vi "Do.vi"(8 "error in":errorcluster, 10 "Actor in":refnum<class "Actor.lvclass">, 11 "Enable Laser Channel 0":refnum<class "Update PAS Laser 0 Enable State MSG.lvclass">) -> (0 "error out":errorcluster, 2 "Actor out":refnum<class "Actor.lvclass">)   [LabVIEW 2016, in "Controller.lvlib" / "Update PAS Laser 0 Enable State MSG.lvclass"]
doc: "(<B>Filename</B>: Actor Framework.lvlib:Message.lvclass:Do.vi)\n\nDefines what a message does when it is received by an actor. Generally, a message instructs an actor to invoke one of its methods. By default, this method does nothing. A child class must override it to define behavior. Create a child class by using the Actor Framework Message Maker dialog box."
uses:
  Update PAS Laser 0 Enable State MSG.lvclass
  G:/sw_repo/For Builds/Nicholas/Controller/Messages/Generic Boolean MSG/Generic Boolean Message.lvclass
  <vilib>/ActorFramework/Actor/Actor.lvclass
  Generic Boolean MSG/Generic Boolean Message.lvclass/Generic Boolean Message.ctl
  Generic Boolean MSG/Read Bool.vi
  <vilib>/rvi/errors/niLvFpgaAdjustHostInterfaceError.vi
  <vilib>/Utility/error.llb/Error Cluster From Error Code.vi
  FPGA Ref.ctl
  <vilib>/rvi/interface/nirviReadWriteControl/nirviReadWriteControl.xnode
  FPGA Bitfiles/serverv4.lvbitx
  gController.lvclass
  NiFpgaLv.dll
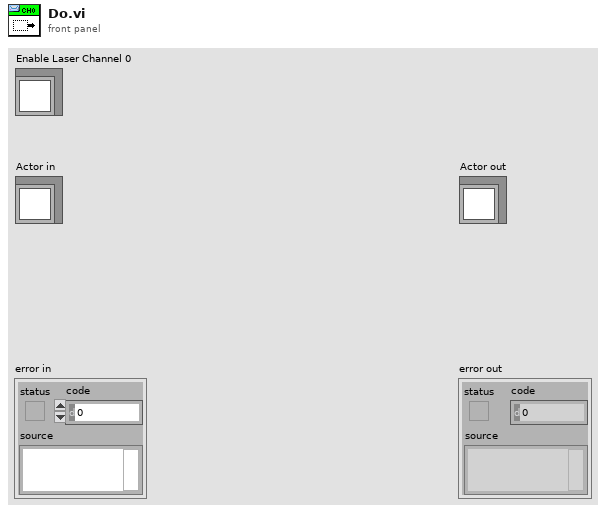
[diagram p1: front panel]
types:
  T1 = typedef "FPGA Ref.ctl" = refnum<k20>
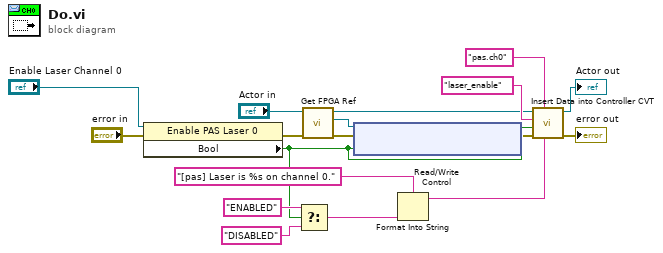
[diagram p0: block diagram]
diagram:
  n1 = property class="Enable PAS Laser 0"(reference="Enable Laser Channel 0", error in="error in") -> (error out=w4:errorcluster, "Bool"=w5:bool)  [unwired: 1 out]
  n2 = Select(t="ENABLED", s=w5, f="DISABLED") -> (s? t:f=w11:string)
  n3 = call "Get FPGA Ref.vi"("error in (no error)"=w4, "Actor In"="Actor in") -> ("error out"=w3:errorcluster, "FPGA Ref"=w6:T1, "Actor Out"=w7:refnum<class "Actor.lvclass">)  [unwired: 7 in]
  n4 = xnode "Read/Write Control"("FPGA VI Reference In"=w6, "error in"=w3, "PAS Laser 1 Enable"=w5) -> ("error out"=w2:errorcluster)  [unwired: 1 out]
  n5 = Format Into String(format string="[pas] Laser is %s on channel 0.", w11) -> (resulting string=w9:string)  [unwired: 2 in, 1 out]
  n6 = call "Insert Data into Controller CVT.vi"("Update MSG"=w9, "Group"="pas.ch0", "error in"=w2, "Data"=w5, "tag"="laser_enable", "Actor in"=w7) -> ("error out"=→"error out":errorcluster, "Actor Out"=→"Actor out":refnum<class "Actor.lvclass">)  [unwired: 4 in]
